vi "LuaVIEW Retrieve Scripts_srv.vi"(7 "certificate":string, 11 "identifier":string) -> (4 "script infos":T1[](array[typedef]), 8 "script errors":cluster{"line numbers":i32[]}[](array[cluster]), 15 "error out":errorcluster)   [LabVIEW 2012]
uses:
  typedefs/clusters/LuaVIEW Script Info.ctl
  clientsrv/typedefs/t_ClientSrv Access Levels.ctl
  typedefs/t_LuaVIEW Task List Methods.ctl
  typedefs/t_LuaVIEW Task State Methods.ctl
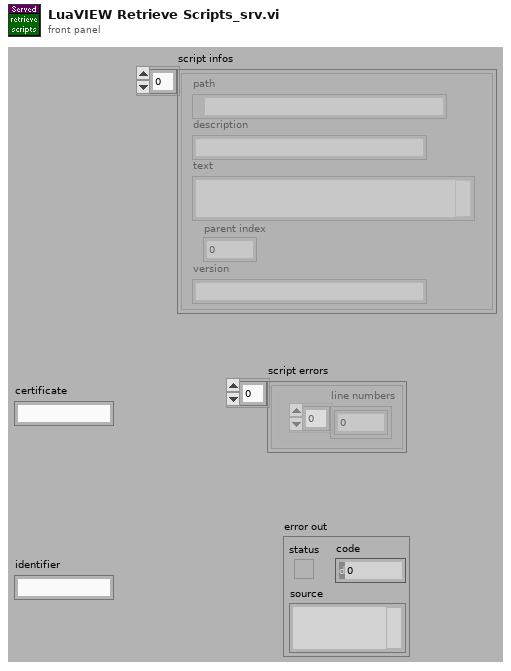
[diagram p1: front panel]
types:
  T1 = typedef "LuaVIEW Script Info.ctl" = cluster{"path":path, "description":string, "text":string, "parent index":i32, "version":string}
  T2 = typedef "t_ClientSrv Access Levels.ctl" = enum16{"observer", "operator", "local"}
  T3 = typedef "t_LuaVIEW Task List Methods.ctl" = enum16{"clear list", "add", "test", "remove", "get ref", "get task info", "get list", "get script info", "ongoing?", "resume", "pause", "stop", "confirm", "message"}
  T4 = typedef "t_LuaVIEW Task State Methods.ctl" = enum16{"cleanup", "set initial", "set mode", "set active mode", "set error", "get task info", "get script info", "set signal", "clear signal", "test handled", "test delegated", "test signal", "handle signal", "delegate signal", "allow signal", "disallow signal", "disallow all", "signals?", "delegated signals?", "protection++", "protection--", "protection=0", "message", "next message", "pop message", "message available?", "force stop", "set swap preps", "apply swap preps"}
  T5 = typedef "t_LuaVIEW Task State Pane.ctl" = refnum<vi>
  T6 = typedef "LuaVIEW Task Info.ctl" = cluster{"main script":string, "identifier":string, "class":string, "description":string, "mode":T7, "handler":string, "LuaVIEW reference":T8, "scripts":i32, "hide":bool, "active":bool, "error msg":string, "defer":bool, "launch":enum16{"asynchronous", "manual", "synchronous"}, "main path valid":bool, "start time":dbl, "swap time":dbl, "task VI":refnum<vi>, "prefsys":enum32{"invalid execution system", "user interface", "standard", "instrument i/o", "data acquisition", "other 1", "other 2", "same as caller"}, "priority":enum32{"invalid priority", "background priority", "normal priority", "above normal priority", "high priority", "time critical priority", "subroutine"}, "signal flags":u32, "allow mask":u32, "handle mask":u32, "disallow manual":bool}
  T7 = typedef "t_LuaVIEW Task Modes.ctl" = enum16{"initializing", "running", "executing", "paused", "error", "swapping"}
  T8 = typedef "t_LuaVIEW Reference.ctl" = refnum<k1>
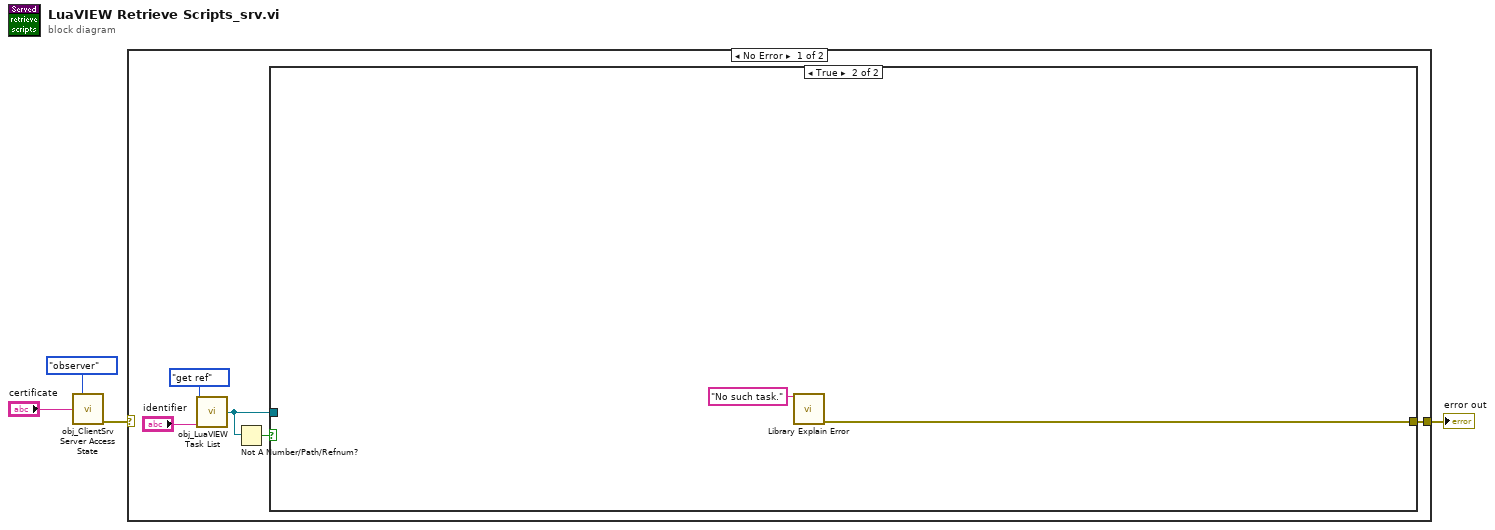
[diagram p0: block diagram]
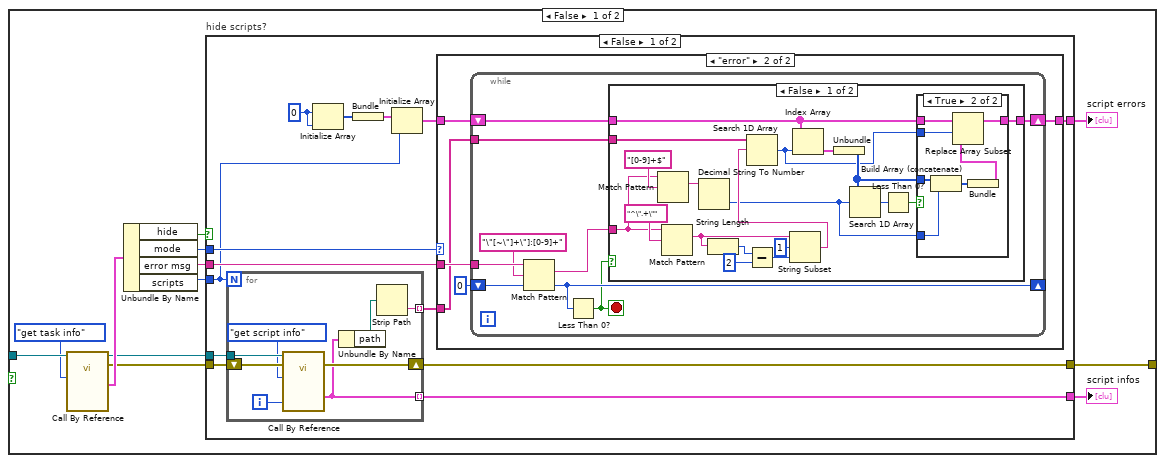
[diagram p2: hidden frame]
diagram:
  n1 = call "obj_ClientSrv Server Access State.vi"("access level"=t_ClientSrv_Access_Levels."observer", "certificate in"="certificate") -> ("error out"=w2:errorcluster)  [unwired: 11 in, 2 out]
  n2 = case shown="No Error" w2 {
    selector: w2 -> [_ w89]
    tunnel: [w5 w89] -> w1
    frame No Error {
      n3 = call "obj_LuaVIEW Task List.vi"("method"=t_LuaVIEW_Task_List_Methods."get ref", "task identifier"="identifier") -> ("state object ref out"=w7:T5)  [unwired: 8 in, 5 out]
      n4 = Not A Number/Path/Refnum?(number/path/refnum=w7) -> (NaN/Path/Refnum?=w6:bool)
      n5 = case shown="True" w6 {
        tunnel: w7 -> [w21 _]
        tunnel: [w17 w87] -> w5
        frame False {
          n6 = call-by-ref "?"(reference=w21, "method"=t_LuaVIEW_Task_State_Methods."get task info") -> (reference out=w16:T5, error out=w18:errorcluster, "task info {get task info}"=w19:T6)  [unwired: 11 in, 4 out]
          n7 = Unbundle By Name(w19) -> ("hide"=w10:bool, "mode"=w13:T7, "error msg"=w14:string, "scripts"=w12:i32)
          n8 = case "hide scripts?" shown="False" w10 {
            tunnel: w18 -> [w34 w86]
            tunnel: [w33 w86] -> w17
            tunnel: w16 -> [w32 _]
            tunnel: [w31 _] -> w15
            tunnel: w14 -> [w30 _]
            tunnel: w13 -> [w28 _]
            tunnel: w12 -> [w24 _]
            tunnel: [w22 _] -> w11
            frame False {
              w27 = 0
              n9 = for {
                N: w24 -> [_]
                shift-right: [w82] -> w33
                shift-left: w34 -> [w85]
                tunnel: w32 -> [w84]
                tunnel: [w80] -> w31 mode=indexing
                tunnel: [w78] -> w29 mode=indexing
                i -> [w81]
                n10 = call-by-ref "?"(reference=w84, error in=w85, "method"=t_LuaVIEW_Task_State_Methods."get script info", "script index"=w81) -> (error out=w82:errorcluster, "script info"=w80:T1)  [unwired: 9 in, 5 out]
                n11 = Unbundle By Name(w80) -> ("path"=w79:path)
                n12 = Strip Path(path=w79) -> (name=w78:string)  [unwired: 1 out]
              }
              n13 = Initialize Array(w27, w27) -> (w26:i32[])
              n14 = Bundle(w26) -> (w25:cluster{i32[]})  [unwired: 1 in]
              n15 = Initialize Array(w25, w24) -> (w23:cluster{i32[]}[])
              n16 = case shown="\"error\"" w28 {
                tunnel: w30 -> [_ w39]
                tunnel: w29 -> [_ w36]
                tunnel: w23 -> [w35 w38]
                tunnel: [w35 w37] -> w22
                frame Default {
                }
                frame "error" {
                  n17 = while {
                    shift-right: [w46] -> _
                    shift-left: 0 -> [w48]
                    tunnel: w39 -> [w49]
                    shift-right: [w41] -> w37
                    shift-left: w38 -> [w42]
                    tunnel: w36 -> [w43]
                    stop <- w44 stop-if-true
                    n18 = Match Pattern(string=w49, regular expression="\"[~\"]+\"]:[0-9]+", offset (0)=w48) -> (match substring=w45:string, offset past match=w46:i32)  [unwired: 2 out]
                    n19 = Less Than 0?(x=w46) -> (x < 0?=w44:bool)
                    n20 = case shown="False" w44 {
                      tunnel: w45 -> [w65 _]
                      tunnel: w43 -> [w59 _]
                      tunnel: w42 -> [w52 w77]
                      tunnel: [w51 w77] -> w41
                      frame False {
                        n21 = Match Pattern(string=w65, regular expression="[0-9]+$") -> (match substring=w67:string)  [unwired: 1 in, 3 out]
                        n22 = Match Pattern(string=w65, regular expression="^\".+\"") -> (match substring=w64:string)  [unwired: 1 in, 3 out]
                        n23 = Decimal String To Number(string=w67) -> (number=w53:i32)  [unwired: 2 in, 1 out]
                        n24 = String Length(string=w64) -> (length=w62:i32)
                        n25 = Subtract(x=w62, y=2) -> (x-y=w61:i32)
                        n26 = String Subset(string=w64, offset (0)=1, length (rest)=w61) -> (substring=w58:string)
                        n27 = Search 1D Array(1D array=w59, element=w58) -> (index of element=w50:i32)  [unwired: 1 in]
                        n28 = Index Array(array=w52, index=w50) -> (element=w57:cluster{i32[]})
                        n29 = Unbundle(w57) -> (w54:i32[])
                        n30 = Search 1D Array(1D array=w54, element=w53) -> (index of element=w56:i32)  [unwired: 1 in]
                        n31 = Less Than 0?(x=w56) -> (x < 0?=w55:bool)
                        n32 = case shown="True" w55 {
                          tunnel: w54 -> [_ w76]
                          tunnel: w53 -> [_ w75]
                          tunnel: w52 -> [w69 w74]
                          tunnel: [w69 w73] -> w51
                          tunnel: w50 -> [_ w72]
                          frame False {
                          }
                          frame True {
                            n33 = Build Array (concatenate)(w76, w75) -> (w71:i32[])
                            n34 = Bundle(w71) -> (w70:cluster{i32[]})  [unwired: 1 in]
                            n35 = Replace Array Subset(array=w74, new element=w70, index=w72) -> (w73:cluster{i32[]}[])
                          }
                        }
                      }
                      frame True {
                      }
                    }
                  }
                }
              }
            }
            frame True {
            }
          }
          "script infos" <- w15
          "script errors" <- w11
        }
        frame True {
          n36 = call "Library Explain Error.vi"("explanation prefix (none)"="No such task.") -> ("explained error"=w87:errorcluster)  [unwired: 14 in]
        }
      }
    }
    frame Error {
    }
  }
  "error out" <- w1
